vi "Shared Set Object Pointer.vi"(10 "Object Pointer":i64, 11 "Data in":refnum<class "Data.lvclass">) -> (3 "Data out":refnum<class "Data.lvclass">)   [LabVIEW 2015, in "MDSplus.lvlib" / "Data.lvclass"]
uses:
  Data.lvclass
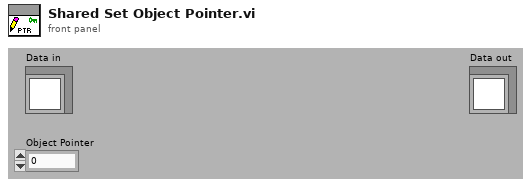
[diagram p1: front panel]
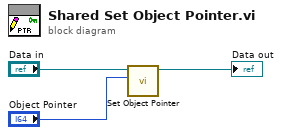
[diagram p0: block diagram]
diagram:
  n1 = call-dynamic "Set Object Pointer.vi"("Object Pointer"="Object Pointer", "Data in"="Data in") -> ("Data out"=→"Data out":refnum<class "Data.lvclass">)  [unwired: 9 in]
